vi "Error Count Channel Names.vi"() -> (3 "error count channel names":string[](array[string]))   [LabVIEW 2020, in "AIM MIL-STD-1553 Scripting.lvlib"]
uses:
  AIM MIL-STD-1553 Scripting.lvlib
  Constants.vi
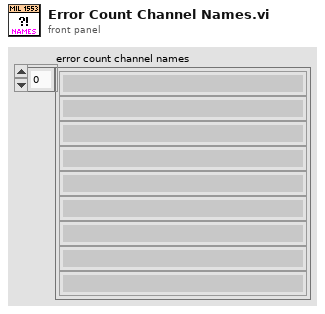
[diagram p1: front panel]
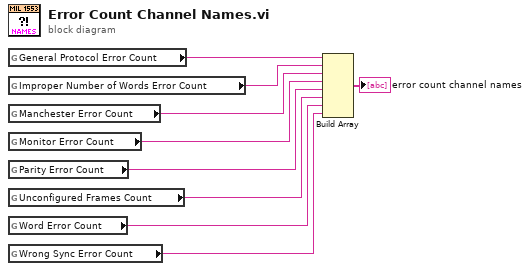
[diagram p0: block diagram]
diagram:
  n1 = global read "Constants.vi" "General Protocol Error Count"() -> (w2:string)
  n2 = global read "Constants.vi" "Improper Number of Words Error Count"() -> (w3:string)
  n3 = global read "Constants.vi" "Manchester Error Count"() -> (w4:string)
  n4 = global read "Constants.vi" "Monitor Error Count"() -> (w5:string)
  n5 = global read "Constants.vi" "Parity Error Count"() -> (w6:string)
  n6 = global read "Constants.vi" "Unconfigured Frames Count"() -> (w7:string)
  n7 = global read "Constants.vi" "Word Error Count"() -> (w8:string)
  n8 = global read "Constants.vi" "Wrong Sync Error Count"() -> (w9:string)
  n9 = Build Array(w2, w3, w4, w5, w6, w7, w8, w9) -> (→"error count channel names":string[])
